vi "Artificial_Pancreas.vi"() -> ()   [LabVIEW 2020]
uses:
  <vilib>/MakerHub/LINX/Public/Peripherals/Analog/Analog Read 1 Chan.vi
  <vilib>/MakerHub/LINX/Public/Peripherals/Digital/Digital Write 1 Chan.vi
  <vilib>/MakerHub/LINX/Public/Peripherals/Analog/Analog Read N Chans.vi
  <vilib>/MakerHub/LINX/Public/Peripherals/Digital/Digital Write N Chans.vi
  <vilib>/MakerHub/LINX/Private/Local IO/LinxAnalogRead.vi
  <vilib>/MakerHub/LINX/Public/Utilities/Check Channel.vi
  <vilib>/MakerHub/LINX/Private/Local IO/LinxDigitalWrite.vi
  <vilib>/MakerHub/LINX/Public/Utilities/Open Serial.vi
  <vilib>/MakerHub/LINX/Private/Utilties/Generate Error.vi
  <vilib>/Waveform/WDTFileIO.llb/Export Waveform To Spreadsheet File.vi
  <vilib>/MakerHub/LINX/LMH-LINX.lvlib
panel:
  in  "file path (dialog if empty)":path=path "C:/Users/User/Desktop/Programs/LabVIEW/LabVIEW_ARDUINO/Data.txt"
  out "Tap water":bool
  out "Salt water":bool
  in  "Tap water":bool
  in  "V high":dbl=2.8
  in  "Salt water":bool
  out "Waveform Chart":dbl(graph)=4.4970703125
  in  "V low":dbl=2.5
  out "Voltage":dbl=4.4970703125
  in  "stop":bool
  in  "Baud Rate Override":u32=115200
  in  "Serial Port":refnum<visa-resource-name>="COM3"
  # "Salt water"
  # "Tap water"
  # "Sensor voltage"
  # "V high"
  # "Serial Port"
  # "V low"
  # "Baud Rate"
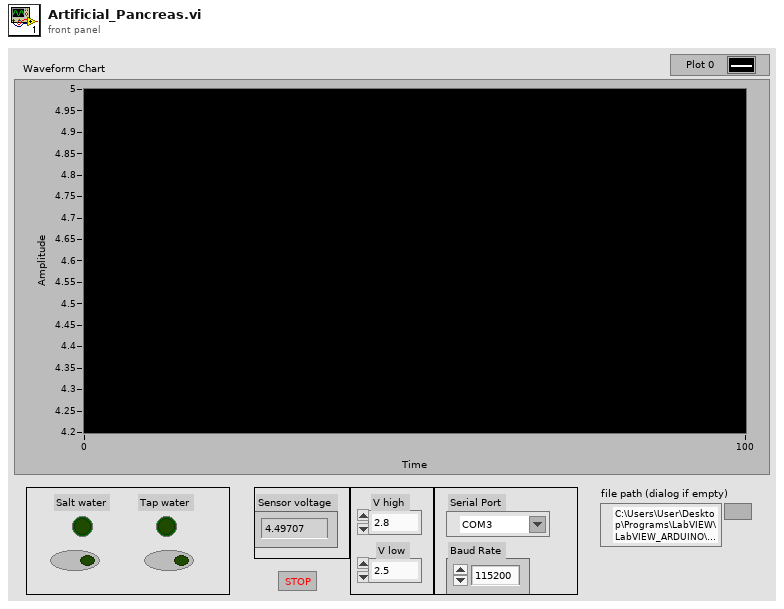
[diagram p1: front panel]
types:
  T1 = typedef "LMH-LINX.lvlib/LINX Ref.ctl" = cluster{"IO":T2, "Interface":T3, "LINX Device Config":T4}
  T2 = typedef "LMH-LINX.lvlib/Platform.ctl" = enum16{"Remote", "Local"}
  T3 = typedef "LMH-LINX.lvlib/Interface.ctl" = enum16{"Serial", "TCP"}
  T4 = typedef "LMH-LINX.lvlib/Device.lvlib/LINX Device Config.ctl" = cluster{"Interface":T3, "COM Port":refnum<visa-resource-name>, "TCP Configuration":T5, "Device Family":u8, "Device ID":u8, "Device Name":string, "TCP Ref":refnum<k5>, "Channels":T6}
  T5 = typedef "LMH-LINX.lvlib/Device.lvlib/TCP Config.ctl" = cluster{"IP Address":string, "Port":u16}
  T6 = typedef "LMH-LINX.lvlib/Channels.ctl" = cluster{"DI":u8[], "DO":u8[], "AI":u8[], "AO":u8[], "PWM":u8[], "QE":u8[], "UART":u8[], "I2C 2":u8[], "SPI":u8[], "CAN":u8[], "Servo":u8[], "AI Ref (V)":dbl, "AI Resolution (Bits)":u8, "AO Ref (V)":dbl, "AO Resolution (Bits)":u8}
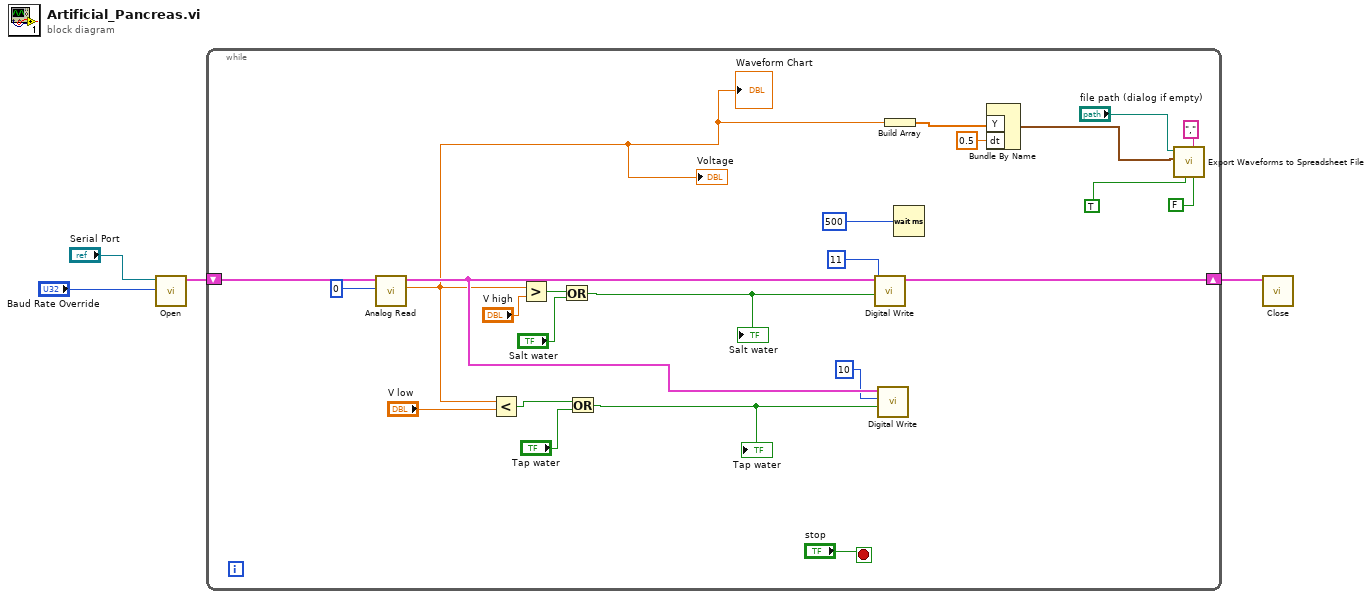
[diagram p0: block diagram]
diagram:
  n1 = call-poly <vilib>:"Open.vi"("Baud Rate Override"="Baud Rate Override", "Serial Port"="Serial Port") -> ("LINX Resource"=w2:T1)  [unwired: 7 in, 2 out]
  n2 = while {
    shift-right: [w24] -> w1
    shift-left: w2 -> [w27]
    stop <- "stop" stop-if-true
    n3 = call-poly <vilib>:"Analog Read.vi"("Analog Channel"=u8 0, "LINX Resource"=w27) -> ("Voltage"=w13:dbl, "LINX Resource"=w19:T1)  [unwired: 6 in, 2 out]
    "Voltage" <- w13
    "Waveform Chart" <- w13
    n4 = Less?(x=w13, y="V low") -> (x < y?=w18:bool)
    n5 = Greater?(x=w13, y="V high") -> (0:w21:bool)
    n6 = Or(x=w21, y="Salt water") -> (x .or. y?=w14:bool)
    "Salt water" <- w14
    n7 = Or(x=w18, y="Tap water") -> (x .or. y?=w15:bool)
    "Tap water" <- w15
    n8 = call-poly <vilib>:"Digital Write.vi"("Output Value"=w14, "DO Channel"=u8 11, "LINX Resource"=w19) -> ("LINX Resource"=w24:T1)  [unwired: 7 in, 1 out]
    n9 = call-poly <vilib>:"Digital Write.vi"("Output Value"=w15, "DO Channel"=u8 10, "LINX Resource"=w19) -> ()  [unwired: 7 in, 2 out]
    n10 = Build Array(w13) -> (w12:dbl[])
    n11 = Wait (ms)(milliseconds to wait=u32 500) -> ()  [unwired: 1 out]
    n12 = Bundle By Name("Y"=w12, "dt"=0.5) -> (w11:waveform(dbl))  [unwired: 1 in]
    n13 = call-poly <vilib>:"Export Waveforms to Spreadsheet File.vi"("header? (write header:T)"=FALSE, "delimiter (Tab)"=",", "append to file? (new file:F)"=TRUE, "waveform"=w11, "file path (dialog if empty)"="file path (dialog if empty)") -> ()  [unwired: 5 in, 2 out]
  }
  n14 = call <vilib>:"Close.vi"("LINX Resource"=w1) -> ()  [unwired: 10 in, 1 out]
